vi "ZMC Search And Open Eth.vi"(8 "error in (no error)":errorcluster caption="错误输入（无错误）", 9 "phandle":u32, 10 "uims":u32, 11 "ipaddr":string) -> (0 "error out":errorcluster caption="错误输出", 1 "phandle out":u32, 2 "function return":i32, 3 "ipaddr out":string)   [LabVIEW 2015, in "zauxdll.lvlib"]
doc: "int32 __stdcall ZMC_SearchAndOpenEth(char *ipaddr, uint32 uims, ZMC_HANDLE * phandle);"
uses:
  zauxdll.lvlib
  zmotion.dll
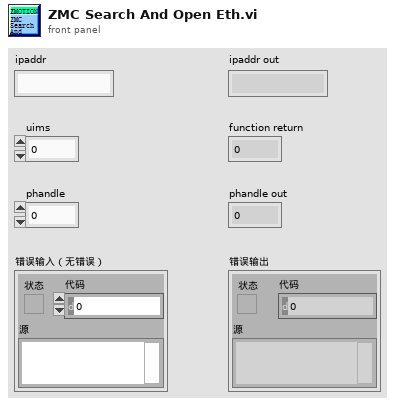
[diagram p1: front panel]
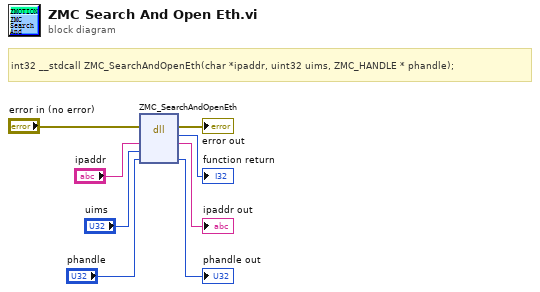
[diagram p0: block diagram]
diagram:
  # "int32 __stdcall ZMC_SearchAndOpenEth(char *ipaddr, uint32 uims, ZMC_HANDLE * phandle);"
  n1 = dll-call lib="C:/Users/VIC/Desktop/GOGORO_SA/system/LLB/zmotion/zaux/zmotion.*" fn="ZMC_SearchAndOpenEth"(error in="error in (no error)", "ipaddr"="ipaddr", "uims"="uims", "phandle"="phandle") -> (error out=→"error out":errorcluster, →"function return":i32, "ipaddr"=→"ipaddr out":string, "phandle"=→"phandle out":u32)  [unwired: 3 in, 1 out]
